vi "Plot Data.vi"(0 "Plots Refnums":T9, 7 "Measurement":T5, 11 "error in (no error)":errorcluster) -> (15 "error out":errorcluster)   [LabVIEW 2014]
uses:
  PlotData Refnums.ctl
  Chooseplot.ctl
  Electrical Data Plot Refnums.ctl
  Optical Spectrum Plot Refnum.ctl
  Measurement.ctl
  WhichInstrument.ctl
  Hardware Control/Parameter Analyzer/Electrical Data.ctl
  Hardware Control/Spectrometer/Spectral Data.ctl
  Hardware Control/Parameter Analyzer/Voltage Plot.ctl
  Hardware Control/Parameter Analyzer/Current Plot.ctl
panel:
  out "PlotData - Choose Plot":T1
  in  "PlotData - Electrical Plot List":T2(tab)
  out "PlotData - Current Plot":cluster{"Time":dbl[], "SMU4":dbl[]}[](graph)=[{"Time"=[0.0, 0.30000000000000004, 0.6000000000000001, 0.9, 1.2000000000000002, 1.5, 1.8, 2.1, 2.4000000000000004, 2.7, 3.0, 3.3000000000000003, 3.6, 3.9000000000000004, 4.2, 4.5, 4.800000000000001, 5.1000000000000005, 5.4, 5.7, 6.0, 6.300000000000001, 6.6000000000000005, 6.9, 7.2, 7.5, 7.800000000000001, 8.1, 8.4, 8.700000000000001, 9.0, 9.3, 9.600000000000001, 9.9, 10.200000000000001, 10.5, 10.8, 11.100000000000001, 11.4, 11.700000000000001, 12.0, 12.3, 12.600000000000001, 12.9, 13.200000000000001, 13.5, 13.8, 14.100000000000001, 14.4, 14.700000000000001, 15.0, 15.3, 15.600000000000001, 15.9, 16.2, 16.5, 16.8, 17.1, 17.400000000000002, 17.7], "SMU4"=[9.99995e-06, 9.99995e-06, 9.99995e-06, 9.99997e-06, 9.99997e-06, 9.99997e-06, 9.99997e-06, 9.999980000000001e-06, 9.99997e-06, 9.999980000000001e-06, 9.99997e-06, 9.999980000000001e-06, 9.99997e-06, 9.99997e-06, 9.99997e-06, 9.99996e-06, 9.99996e-06, 9.99996e-06, 9.99996e-06, 9.99997e-06, 9.99997e-06, 9.999980000000001e-06, 9.99997e-06, 9.99997e-06, 9.99997e-06, 9.99997e-06, 9.99997e-06, 9.999980000000001e-06, 9.999980000000001e-06, 9.99996e-06, 9.99997e-06, 9.99996e-06, 9.99997e-06, 9.99997e-06, 9.99997e-06, 9.99997e-06, 9.999980000000001e-06, 9.99997e-06, 9.999980000000001e-06, 9.999980000000001e-06, 9.99997e-06, 9.99997e-06, 9.99997e-06, 9.99996e-06, 9.99996e-06, 9.99997e-06, 9.99997e-06, 9.99996e-06, 9.99996e-06, 9.99997e-06, 9.99997e-06, 9.99997e-06, 9.99997e-06, 9.99997e-06, 9.99996e-06, 9.99997e-06, 9.99997e-06, 9.99997e-06, 9.99997e-06, 9.99996e-06]}, {"Time"=[0.0, 0.30000000000000004, 0.6000000000000001, 0.9, 1.2000000000000002, 1.5, 1.8, 2.1, 2.4000000000000004, 2.7, 3.0, 3.3000000000000003, 3.6, 3.9000000000000004, 4.2, 4.5, 4.800000000000001, 5.1000000000000005, 5.4, 5.7, 6.0, 6.300000000000001, 6.6000000000000005, 6.9, 7.2, 7.5, 7.800000000000001, 8.1, 8.4, 8.700000000000001, 9.0, 9.3, 9.600000000000001, 9.9, 10.200000000000001, 10.5, 10.8, 11.100000000000001, 11.4, 11.700000000000001, 12.0, 12.3, 12.600000000000001, 12.9, 13.200000000000001, 13.5, 13.8, 14.100000000000001, 14.4, 14.700000000000001, 15.0, 15.3, 15.600000000000001, 15.9, 16.2, 16.5, 16.8, 17.1, 17.400000000000002, 17.7], "SMU4"=[-1.00004e-05, -1.000039e-05, -1.000039e-05, -1.0000409999999999e-05, -1.000039e-05, -1.000039e-05, -1.00004e-05, -1.000043e-05, -1.000042e-05, -1.0000409999999999e-05, -1.000039e-05, -1.000039e-05, -1.0000409999999999e-05, -1.00004e-05, -1.000038e-05, -1.000038e-05, -1.000039e-05, -1.000037e-05, -1.000038e-05, -1.000039e-05, -1.000039e-05, -1.000039e-05, -1.000039e-05, -1.000039e-05, -1.00004e-05, -1.000037e-05, -1.000038e-05, -1.000039e-05, -1.00004e-05, -1.00004e-05, -1.00004e-05, -1.000037e-05, -1.000037e-05, -1.000037e-05, -1.000036e-05, -1.000039e-05, -1.000038e-05, -1.000037e-05, -1.000036e-05, -1.000037e-05, -1.000038e-05, -1.000037e-05, -1.000038e-05, -1.000036e-05, -1.000037e-05, -1.000037e-05, -1.000037e-05, -1.000039e-05, -1.000038e-05, -1.000036e-05, -1.000037e-05, -1.000039e-05, -1.000036e-05, -1.000037e-05, -1.000038e-05, -1.00004e-05, -1.0000409999999999e-05, -1.000038e-05, -1.000038e-05, -1.00004e-05]}]
  out "PlotData - Voltage Plot":cluster{"Time":dbl[], "SMU4":dbl[]}[](graph)=[{"Time"=[0.0, 0.30000000000000004, 0.6000000000000001, 0.9, 1.2000000000000002, 1.5, 1.8, 2.1, 2.4000000000000004, 2.7, 3.0, 3.3000000000000003, 3.6, 3.9000000000000004, 4.2, 4.5, 4.800000000000001, 5.1000000000000005, 5.4, 5.7, 6.0, 6.300000000000001, 6.6000000000000005, 6.9, 7.2, 7.5, 7.800000000000001, 8.1, 8.4, 8.700000000000001, 9.0, 9.3, 9.600000000000001, 9.9, 10.200000000000001, 10.5, 10.8, 11.100000000000001, 11.4, 11.700000000000001, 12.0, 12.3, 12.600000000000001, 12.9, 13.200000000000001, 13.5, 13.8, 14.100000000000001, 14.4, 14.700000000000001, 15.0, 15.3, 15.600000000000001, 15.9, 16.2, 16.5, 16.8, 17.1, 17.400000000000002, 17.7], "SMU4"=[9.99995e-06, 9.99995e-06, 9.99995e-06, 9.99997e-06, 9.99997e-06, 9.99997e-06, 9.99997e-06, 9.999980000000001e-06, 9.99997e-06, 9.999980000000001e-06, 9.99997e-06, 9.999980000000001e-06, 9.99997e-06, 9.99997e-06, 9.99997e-06, 9.99996e-06, 9.99996e-06, 9.99996e-06, 9.99996e-06, 9.99997e-06, 9.99997e-06, 9.999980000000001e-06, 9.99997e-06, 9.99997e-06, 9.99997e-06, 9.99997e-06, 9.99997e-06, 9.999980000000001e-06, 9.999980000000001e-06, 9.99996e-06, 9.99997e-06, 9.99996e-06, 9.99997e-06, 9.99997e-06, 9.99997e-06, 9.99997e-06, 9.999980000000001e-06, 9.99997e-06, 9.999980000000001e-06, 9.999980000000001e-06, 9.99997e-06, 9.99997e-06, 9.99997e-06, 9.99996e-06, 9.99996e-06, 9.99997e-06, 9.99997e-06, 9.99996e-06, 9.99996e-06, 9.99997e-06, 9.99997e-06, 9.99997e-06, 9.99997e-06, 9.99997e-06, 9.99996e-06, 9.99997e-06, 9.99997e-06, 9.99997e-06, 9.99997e-06, 9.99996e-06]}, {"Time"=[0.0, 0.30000000000000004, 0.6000000000000001, 0.9, 1.2000000000000002, 1.5, 1.8, 2.1, 2.4000000000000004, 2.7, 3.0, 3.3000000000000003, 3.6, 3.9000000000000004, 4.2, 4.5, 4.800000000000001, 5.1000000000000005, 5.4, 5.7, 6.0, 6.300000000000001, 6.6000000000000005, 6.9, 7.2, 7.5, 7.800000000000001, 8.1, 8.4, 8.700000000000001, 9.0, 9.3, 9.600000000000001, 9.9, 10.200000000000001, 10.5, 10.8, 11.100000000000001, 11.4, 11.700000000000001, 12.0, 12.3, 12.600000000000001, 12.9, 13.200000000000001, 13.5, 13.8, 14.100000000000001, 14.4, 14.700000000000001, 15.0, 15.3, 15.600000000000001, 15.9, 16.2, 16.5, 16.8, 17.1, 17.400000000000002, 17.7], "SMU4"=[-1.00004e-05, -1.000039e-05, -1.000039e-05, -1.0000409999999999e-05, -1.000039e-05, -1.000039e-05, -1.00004e-05, -1.000043e-05, -1.000042e-05, -1.0000409999999999e-05, -1.000039e-05, -1.000039e-05, -1.0000409999999999e-05, -1.00004e-05, -1.000038e-05, -1.000038e-05, -1.000039e-05, -1.000037e-05, -1.000038e-05, -1.000039e-05, -1.000039e-05, -1.000039e-05, -1.000039e-05, -1.000039e-05, -1.00004e-05, -1.000037e-05, -1.000038e-05, -1.000039e-05, -1.00004e-05, -1.00004e-05, -1.00004e-05, -1.000037e-05, -1.000037e-05, -1.000037e-05, -1.000036e-05, -1.000039e-05, -1.000038e-05, -1.000037e-05, -1.000036e-05, -1.000037e-05, -1.000038e-05, -1.000037e-05, -1.000038e-05, -1.000036e-05, -1.000037e-05, -1.000037e-05, -1.000037e-05, -1.000039e-05, -1.000038e-05, -1.000036e-05, -1.000037e-05, -1.000039e-05, -1.000036e-05, -1.000037e-05, -1.000038e-05, -1.00004e-05, -1.0000409999999999e-05, -1.000038e-05, -1.000038e-05, -1.00004e-05]}]
  out "PlotData - dI/dV-V Characteristic":cluster{"V3":dbl[], "I1":dbl[]}[](graph) caption="Differential Resistance"
  out "PlotData - IV Characteristic":cluster{"V3":dbl[], "I1":dbl[]}[](graph) caption="Current Voltage Characteristic"
  in  "PlotData - Optical Spectra":enum32{"Energy", "Wavelength", "Raman Shift"}(tab)
  out "Optical Spectrum vs Energy":cluster{"data":dbl[], "data":dbl[]}(graph)
  out "Optical Spectrum vs Wavelength":cluster{"data":dbl[], "data":dbl[]}(graph)
  out "Optical Spectrum vs Raman Shift":cluster{"data":dbl[], "data":dbl[]}(graph)
  in  "Optoelectronic Spectrum":enum32{"Energy", "Wavelength", "Raman Shift"}(tab)
  out "Optoelectronic Spectrum vs Energy":cluster{"data":dbl[], "data":dbl[]}(graph)
  out "Optoelectronic Spectrum vs Wavelength":cluster{"data":dbl[], "data":dbl[]}(graph)
  out "Optoelectronic Spectrum vs Raman Shift":cluster{"data":dbl[], "data":dbl[]}(graph)
  out "Optoelectronic Voltage Trace":T3=[{"Time"=[0.0, 0.30000000000000004, 0.6000000000000001, 0.9, 1.2000000000000002, 1.5, 1.8, 2.1, 2.4000000000000004, 2.7, 3.0, 3.3000000000000003, 3.6, 3.9000000000000004, 4.2, 4.5, 4.800000000000001, 5.1000000000000005, 5.4, 5.7, 6.0, 6.300000000000001, 6.6000000000000005, 6.9, 7.2, 7.5, 7.800000000000001, 8.1, 8.4, 8.700000000000001, 9.0, 9.3, 9.600000000000001, 9.9, 10.200000000000001, 10.5, 10.8, 11.100000000000001, 11.4, 11.700000000000001, 12.0, 12.3, 12.600000000000001, 12.9, 13.200000000000001, 13.5, 13.8, 14.100000000000001, 14.4, 14.700000000000001, 15.0, 15.3, 15.600000000000001, 15.9, 16.2, 16.5, 16.8, 17.1, 17.400000000000002, 17.7], "SMU4"=[9.99995e-06, 9.99995e-06, 9.99995e-06, 9.99997e-06, 9.99997e-06, 9.99997e-06, 9.99997e-06, 9.999980000000001e-06, 9.99997e-06, 9.999980000000001e-06, 9.99997e-06, 9.999980000000001e-06, 9.99997e-06, 9.99997e-06, 9.99997e-06, 9.99996e-06, 9.99996e-06, 9.99996e-06, 9.99996e-06, 9.99997e-06, 9.99997e-06, 9.999980000000001e-06, 9.99997e-06, 9.99997e-06, 9.99997e-06, 9.99997e-06, 9.99997e-06, 9.999980000000001e-06, 9.999980000000001e-06, 9.99996e-06, 9.99997e-06, 9.99996e-06, 9.99997e-06, 9.99997e-06, 9.99997e-06, 9.99997e-06, 9.999980000000001e-06, 9.99997e-06, 9.999980000000001e-06, 9.999980000000001e-06, 9.99997e-06, 9.99997e-06, 9.99997e-06, 9.99996e-06, 9.99996e-06, 9.99997e-06, 9.99997e-06, 9.99996e-06, 9.99996e-06, 9.99997e-06, 9.99997e-06, 9.99997e-06, 9.99997e-06, 9.99997e-06, 9.99996e-06, 9.99997e-06, 9.99997e-06, 9.99997e-06, 9.99997e-06, 9.99996e-06]}, {"Time"=[0.0, 0.30000000000000004, 0.6000000000000001, 0.9, 1.2000000000000002, 1.5, 1.8, 2.1, 2.4000000000000004, 2.7, 3.0, 3.3000000000000003, 3.6, 3.9000000000000004, 4.2, 4.5, 4.800000000000001, 5.1000000000000005, 5.4, 5.7, 6.0, 6.300000000000001, 6.6000000000000005, 6.9, 7.2, 7.5, 7.800000000000001, 8.1, 8.4, 8.700000000000001, 9.0, 9.3, 9.600000000000001, 9.9, 10.200000000000001, 10.5, 10.8, 11.100000000000001, 11.4, 11.700000000000001, 12.0, 12.3, 12.600000000000001, 12.9, 13.200000000000001, 13.5, 13.8, 14.100000000000001, 14.4, 14.700000000000001, 15.0, 15.3, 15.600000000000001, 15.9, 16.2, 16.5, 16.8, 17.1, 17.400000000000002, 17.7], "SMU4"=[-1.00004e-05, -1.000039e-05, -1.000039e-05, -1.0000409999999999e-05, -1.000039e-05, -1.000039e-05, -1.00004e-05, -1.000043e-05, -1.000042e-05, -1.0000409999999999e-05, -1.000039e-05, -1.000039e-05, -1.0000409999999999e-05, -1.00004e-05, -1.000038e-05, -1.000038e-05, -1.000039e-05, -1.000037e-05, -1.000038e-05, -1.000039e-05, -1.000039e-05, -1.000039e-05, -1.000039e-05, -1.000039e-05, -1.00004e-05, -1.000037e-05, -1.000038e-05, -1.000039e-05, -1.00004e-05, -1.00004e-05, -1.00004e-05, -1.000037e-05, -1.000037e-05, -1.000037e-05, -1.000036e-05, -1.000039e-05, -1.000038e-05, -1.000037e-05, -1.000036e-05, -1.000037e-05, -1.000038e-05, -1.000037e-05, -1.000038e-05, -1.000036e-05, -1.000037e-05, -1.000037e-05, -1.000037e-05, -1.000039e-05, -1.000038e-05, -1.000036e-05, -1.000037e-05, -1.000039e-05, -1.000036e-05, -1.000037e-05, -1.000038e-05, -1.00004e-05, -1.0000409999999999e-05, -1.000038e-05, -1.000038e-05, -1.00004e-05]}]
  out "Optoelectronic Current Trace":T4=[{"Time"=[0.0, 0.30000000000000004, 0.6000000000000001, 0.9, 1.2000000000000002, 1.5, 1.8, 2.1, 2.4000000000000004, 2.7, 3.0, 3.3000000000000003, 3.6, 3.9000000000000004, 4.2, 4.5, 4.800000000000001, 5.1000000000000005, 5.4, 5.7, 6.0, 6.300000000000001, 6.6000000000000005, 6.9, 7.2, 7.5, 7.800000000000001, 8.1, 8.4, 8.700000000000001, 9.0, 9.3, 9.600000000000001, 9.9, 10.200000000000001, 10.5, 10.8, 11.100000000000001, 11.4, 11.700000000000001, 12.0, 12.3, 12.600000000000001, 12.9, 13.200000000000001, 13.5, 13.8, 14.100000000000001, 14.4, 14.700000000000001, 15.0, 15.3, 15.600000000000001, 15.9, 16.2, 16.5, 16.8, 17.1, 17.400000000000002, 17.7], "SMU4"=[9.99995e-06, 9.99995e-06, 9.99995e-06, 9.99997e-06, 9.99997e-06, 9.99997e-06, 9.99997e-06, 9.999980000000001e-06, 9.99997e-06, 9.999980000000001e-06, 9.99997e-06, 9.999980000000001e-06, 9.99997e-06, 9.99997e-06, 9.99997e-06, 9.99996e-06, 9.99996e-06, 9.99996e-06, 9.99996e-06, 9.99997e-06, 9.99997e-06, 9.999980000000001e-06, 9.99997e-06, 9.99997e-06, 9.99997e-06, 9.99997e-06, 9.99997e-06, 9.999980000000001e-06, 9.999980000000001e-06, 9.99996e-06, 9.99997e-06, 9.99996e-06, 9.99997e-06, 9.99997e-06, 9.99997e-06, 9.99997e-06, 9.999980000000001e-06, 9.99997e-06, 9.999980000000001e-06, 9.999980000000001e-06, 9.99997e-06, 9.99997e-06, 9.99997e-06, 9.99996e-06, 9.99996e-06, 9.99997e-06, 9.99997e-06, 9.99996e-06, 9.99996e-06, 9.99997e-06, 9.99997e-06, 9.99997e-06, 9.99997e-06, 9.99997e-06, 9.99996e-06, 9.99997e-06, 9.99997e-06, 9.99997e-06, 9.99997e-06, 9.99996e-06]}, {"Time"=[0.0, 0.30000000000000004, 0.6000000000000001, 0.9, 1.2000000000000002, 1.5, 1.8, 2.1, 2.4000000000000004, 2.7, 3.0, 3.3000000000000003, 3.6, 3.9000000000000004, 4.2, 4.5, 4.800000000000001, 5.1000000000000005, 5.4, 5.7, 6.0, 6.300000000000001, 6.6000000000000005, 6.9, 7.2, 7.5, 7.800000000000001, 8.1, 8.4, 8.700000000000001, 9.0, 9.3, 9.600000000000001, 9.9, 10.200000000000001, 10.5, 10.8, 11.100000000000001, 11.4, 11.700000000000001, 12.0, 12.3, 12.600000000000001, 12.9, 13.200000000000001, 13.5, 13.8, 14.100000000000001, 14.4, 14.700000000000001, 15.0, 15.3, 15.600000000000001, 15.9, 16.2, 16.5, 16.8, 17.1, 17.400000000000002, 17.7], "SMU4"=[-1.00004e-05, -1.000039e-05, -1.000039e-05, -1.0000409999999999e-05, -1.000039e-05, -1.000039e-05, -1.00004e-05, -1.000043e-05, -1.000042e-05, -1.0000409999999999e-05, -1.000039e-05, -1.000039e-05, -1.0000409999999999e-05, -1.00004e-05, -1.000038e-05, -1.000038e-05, -1.000039e-05, -1.000037e-05, -1.000038e-05, -1.000039e-05, -1.000039e-05, -1.000039e-05, -1.000039e-05, -1.000039e-05, -1.00004e-05, -1.000037e-05, -1.000038e-05, -1.000039e-05, -1.00004e-05, -1.00004e-05, -1.00004e-05, -1.000037e-05, -1.000037e-05, -1.000037e-05, -1.000036e-05, -1.000039e-05, -1.000038e-05, -1.000037e-05, -1.000036e-05, -1.000037e-05, -1.000038e-05, -1.000037e-05, -1.000038e-05, -1.000036e-05, -1.000037e-05, -1.000037e-05, -1.000037e-05, -1.000039e-05, -1.000038e-05, -1.000036e-05, -1.000037e-05, -1.000039e-05, -1.000036e-05, -1.000037e-05, -1.000038e-05, -1.00004e-05, -1.0000409999999999e-05, -1.000038e-05, -1.000038e-05, -1.00004e-05]}]
  # "LICENSED MATERIALS – PROPERTY OF IBM\nCopyright IBM Corp. 2016,\nALL RIGHTS RESERVED"
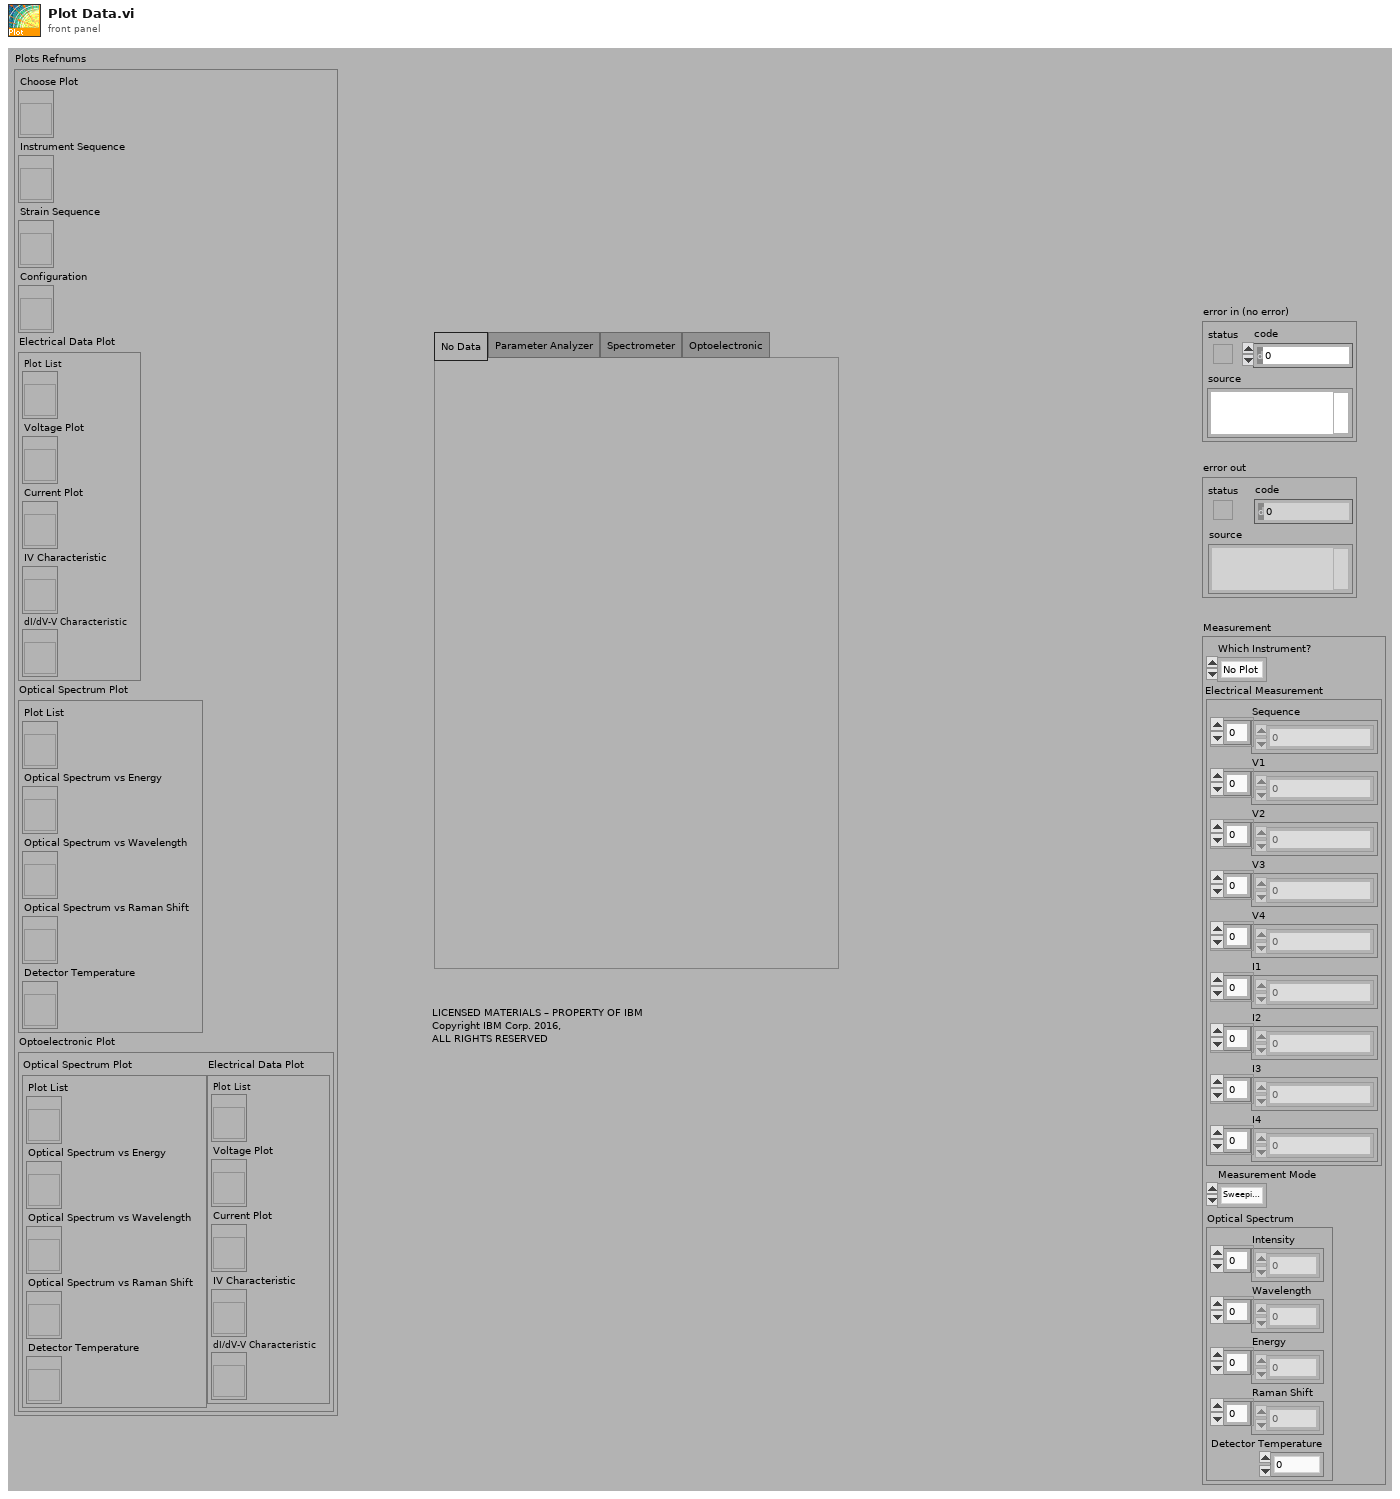
[diagram p1: front panel]
types:
  T1 = typedef "Chooseplot.ctl" = enum32{"No Data", "Parameter Analyzer", "Spectrometer", "Optoelectronic"}
  T2 = enum32{"Current & Voltage Traces", "Four | Two Probe"}
  T3 = typedef "Voltage Plot.ctl" = cluster{"Time":dbl[], "SMU4":dbl[]}[]
  T4 = typedef "Current Plot.ctl" = cluster{"Time":dbl[], "SMU4":dbl[]}[]
  T5 = typedef "Measurement.ctl" = cluster{"Which Instrument?":T6, "Electrical Measurement":T7, "Measurement Mode":enum16{"Sweeping Mode", "Sampling Mode"}, "Optical Spectrum":T8}
  T6 = typedef "WhichInstrument.ctl" = enum16{"No Plot", "Spectrometer", "Parameter Analyzer", "Optoelectronic"}
  T7 = typedef "Electrical Data.ctl" = cluster{"Sequence":dbl[], "V1":dbl[], "V2":dbl[], "V3":dbl[], "V4":dbl[], "I1":dbl[], "I2":dbl[], "I3":dbl[], "I4":dbl[]}
  T8 = typedef "Spectral Data.ctl" = cluster{"Intensity":dbl[], "Wavelength":dbl[], "Energy":dbl[], "Raman Shift":dbl[], "Detector Temperature":dbl}
  T9 = typedef "PlotData Refnums.ctl" = cluster{"Choose Plot":refnum<vi>, "Instrument Sequence":refnum<vi>, "Strain Sequence":refnum<vi>, "Configuration":refnum<vi>, "Electrical Data Plot":T10, "Optical Spectrum Plot":T11, "Optoelectronic Plot":cluster{"Optical Spectrum Plot":T11, "Electrical Data Plot":T10}}
  T10 = typedef "Electrical Data Plot Refnums.ctl" = cluster{"Plot List":refnum<vi>, "Voltage Plot":refnum<vi>, "Current Plot":refnum<vi>, "IV Characteristic":refnum<vi>, "dI/dV-V Characteristic":refnum<vi>}
  T11 = typedef "Optical Spectrum Plot Refnum.ctl" = cluster{"Plot List":refnum<vi>, "Optical Spectrum vs Energy":refnum<vi>, "Optical Spectrum vs Wavelength":refnum<vi>, "Optical Spectrum vs Raman Shift":refnum<vi>, "Detector Temperature":refnum<vi>}
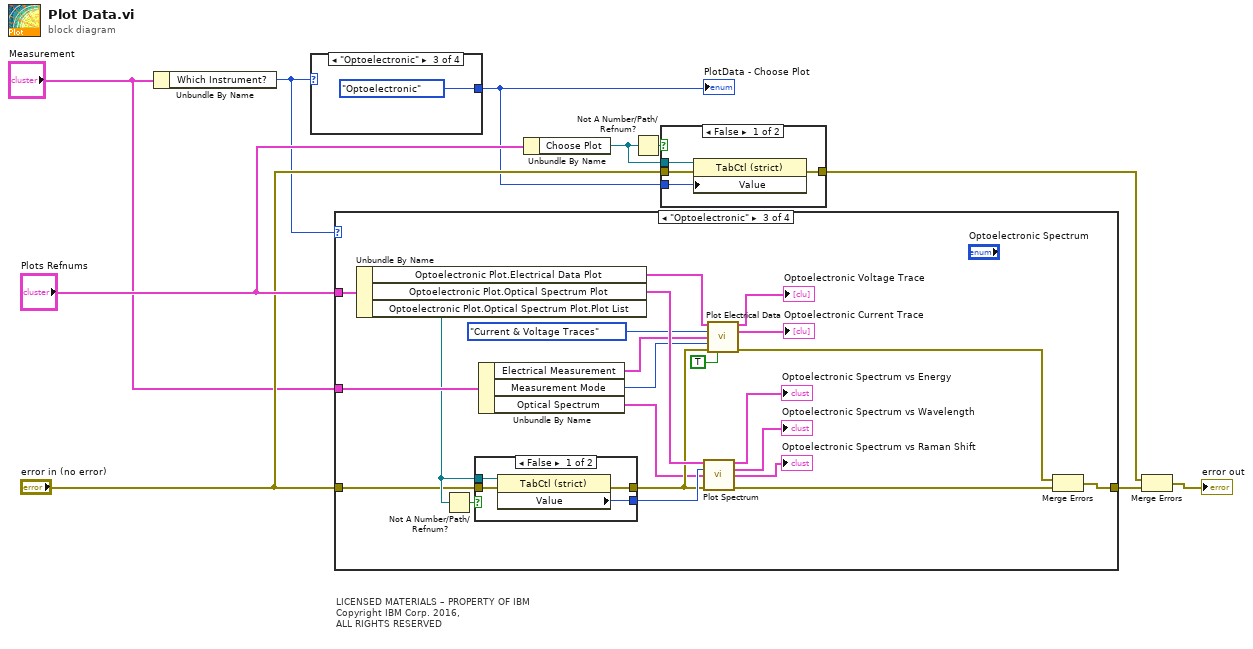
[diagram p0: block diagram]
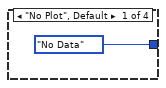
[diagram p2: hidden frame]
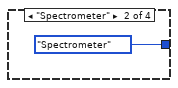
[diagram p3: hidden frame]
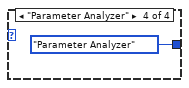
[diagram p4: hidden frame]
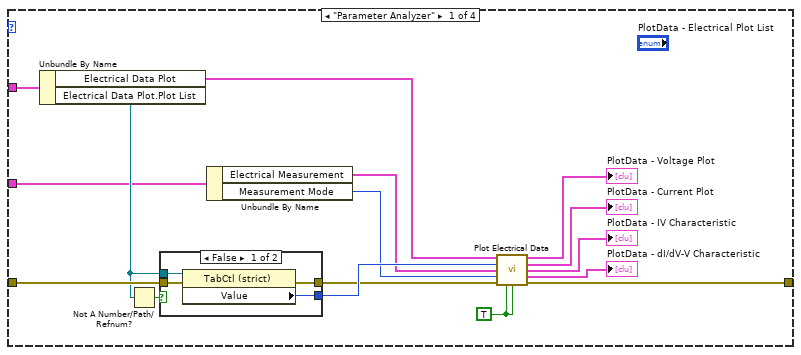
[diagram p6: hidden frame]
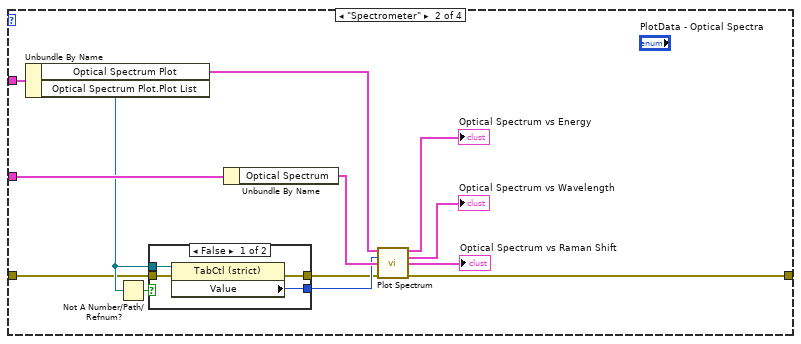
[diagram p8: hidden frame]
diagram:
  # "LICENSED MATERIALS – PROPERTY OF IBM\nCopyright IBM Corp. 2016,\nALL RIGHTS RESERVED"
  n1 = Unbundle By Name("Measurement") -> ("Which Instrument?"=w2:T6)
  n2 = case shown="\"Optoelectronic\"" w2 {
    tunnel: [Chooseplot."No Data" ("PlotData - Choose Plot") Chooseplot."Spectrometer" ("PlotData - Choose Plot") Chooseplot."Optoelectronic" ("PlotData - Choose Plot") Chooseplot."Parameter Analyzer" ("PlotData - Choose Plot")] -> w1
    frame "No Plot", Default {
    }
    frame "Spectrometer" {
    }
    frame "Optoelectronic" {
    }
    frame "Parameter Analyzer" {
    }
  }
  "PlotData - Choose Plot" <- w1
  n3 = case shown="\"Optoelectronic\"" w2 {
    tunnel: [w30 w48 w60 w81] -> w6
    tunnel: "error in (no error)" -> [w26 w40 w69 w81]
    tunnel: "Plots Refnums" -> [w29 w47 w75 _]
    tunnel: "Measurement" -> [w22 w46 w74 _]
    frame "Parameter Analyzer" {
      w19 = TRUE ("Update Pane?")
      n4 = Unbundle By Name(w29) -> ("Electrical Data Plot"=w28:T10, "Electrical Data Plot.Plot List"=w23:refnum<vi>)
      n5 = Not A Number/Path/Refnum?(number/path/refnum=w23) -> (NaN/Path/Refnum?=w24:bool)
      n6 = case shown="False" w24 {
        tunnel: w23 -> [w34 _]
        tunnel: [w33 _] -> w27
        tunnel: w26 -> [w32 w35]
        tunnel: [w31 w35] -> w25
        frame False {
          n7 = property class="TabCtl (strict)"(reference=w34, error in=w32) -> (error out=w31:errorcluster, "Value"=w33:T2)  [unwired: 1 out]
        }
        frame True {
        }
      }
      n8 = Unbundle By Name(w22) -> ("Electrical Measurement"=w21:T7, "Measurement Mode"=w20:enum16{"Sweeping Mode", "Sampling Mode"})
      n9 = call "Plot Electrical Data.vi"("Plot Refnums"=w28, "Plot List"=w27, "Electrical Measurement"=w21, "Measurement Mode"=w20, "error in (no error)"=w25, "Update Labels?"=w19, "Update Pane?"=w19) -> ("Voltage Plot Array"=→"PlotData - Voltage Plot":cluster{"Sequence":dbl[], "Data":dbl[]}[], "Current Plot Array"=→"PlotData - Current Plot":cluster{"Sequence":dbl[], "Data":dbl[]}[], "Current Voltage Array"=→"PlotData - IV Characteristic":cluster{"Voltage":dbl[], "Current":dbl[]}[], "Differential Resistance Array"=→"PlotData - dI/dV-V Characteristic":cluster{"Voltage":dbl[], "Resistance":dbl[]}[], "error out"=w30:errorcluster)  [unwired: 4 out]
    }
    frame "Spectrometer" {
      n10 = Unbundle By Name(w47) -> ("Optical Spectrum Plot"=w44:T11, "Optical Spectrum Plot.Plot List"=w42:refnum<vi>)
      n11 = Not A Number/Path/Refnum?(number/path/refnum=w42) -> (NaN/Path/Refnum?=w43:bool)
      n12 = case shown="False" w43 {
        tunnel: w42 -> [w52 _]
        tunnel: [w51 _] -> w41
        tunnel: w40 -> [w50 w53]
        tunnel: [w49 w53] -> w39
        frame False {
          n13 = property class="TabCtl (strict)"(reference=w52, error in=w50) -> (error out=w49:errorcluster, "Value"=w51:enum32{"Energy", "Wavelength", "Raman Shift"})  [unwired: 1 out]
        }
        frame True {
        }
      }
      n14 = Unbundle By Name(w46) -> ("Optical Spectrum"=w45:T8)
      n15 = call "Plot Spectrum.vi"("Optical Spectrum Plot"=w44, "Optical Spectrum"=w41, "Spectrum"=w45, "error in (no error)"=w39) -> ("Optical Spectrum vs Energy"=→"Optical Spectrum vs Energy":cluster{"data":dbl[], "data":dbl[]}, "Optical Spectrum vs Wavelength"=→"Optical Spectrum vs Wavelength":cluster{"data":dbl[], "data":dbl[]}, "Optical Spectrum vs Raman Shift"=→"Optical Spectrum vs Raman Shift":cluster{"data":dbl[], "data":dbl[]}, "error out"=w48:errorcluster)  [unwired: 8 in]
    }
    frame "Optoelectronic" {
      n16 = Unbundle By Name(w75) -> ("Optoelectronic Plot.Electrical Data Plot"=w62:T10, "Optoelectronic Plot.Optical Spectrum Plot"=w73:T11, "Optoelectronic Plot.Optical Spectrum Plot.Plot List"=w71:refnum<vi>)
      n17 = Not A Number/Path/Refnum?(number/path/refnum=w71) -> (NaN/Path/Refnum?=w72:bool)
      n18 = case shown="False" w72 {
        tunnel: w71 -> [w79 _]
        tunnel: [w78 _] -> w70
        tunnel: w69 -> [w77 w80]
        tunnel: [w76 w80] -> w65
        frame False {
          n19 = property class="TabCtl (strict)"(reference=w79, error in=w77) -> (error out=w76:errorcluster, "Value"=w78:enum32{"Energy", "Wavelength", "Raman Shift"})  [unwired: 1 out]
        }
        frame True {
        }
      }
      n20 = Unbundle By Name(w74) -> ("Electrical Measurement"=w57:T7, "Measurement Mode"=w55:enum16{"Sweeping Mode", "Sampling Mode"}, "Optical Spectrum"=w56:T8)
      n21 = call "Plot Spectrum.vi"("Optical Spectrum Plot"=w73, "Optical Spectrum"=w70, "Spectrum"=w56, "error in (no error)"=w65) -> ("Optical Spectrum vs Energy"=→"Optoelectronic Spectrum vs Energy":cluster{"data":dbl[], "data":dbl[]}, "Optical Spectrum vs Wavelength"=→"Optoelectronic Spectrum vs Wavelength":cluster{"data":dbl[], "data":dbl[]}, "Optical Spectrum vs Raman Shift"=→"Optoelectronic Spectrum vs Raman Shift":cluster{"data":dbl[], "data":dbl[]}, "error out"=w61:errorcluster)  [unwired: 8 in]
      n22 = call "Plot Electrical Data.vi"("Plot Refnums"=w62, "Plot List"=T2."Current & Voltage Traces", "Electrical Measurement"=w57, "Measurement Mode"=w55, "error in (no error)"=w65, "Update Labels?"=TRUE) -> ("Voltage Plot Array"=→"Optoelectronic Voltage Trace":cluster{"Sequence":dbl[], "Data":dbl[]}[], "Current Plot Array"=→"Optoelectronic Current Trace":cluster{"Sequence":dbl[], "Data":dbl[]}[], "error out"=w59:errorcluster)  [unwired: 1 in, 6 out]
      n23 = Merge Errors(w59, w61) -> (w60:errorcluster)
    }
    frame "No Plot", Default {
    }
  }
  n24 = Unbundle By Name("Plots Refnums") -> ("Choose Plot"=w4:refnum<vi>)
  n25 = Not A Number/Path/Refnum?(number/path/refnum=w4) -> (NaN/Path/Refnum?=w5:bool)
  n26 = case shown="False" w5 {
    tunnel: w4 -> [w85 _]
    tunnel: "error in (no error)" -> [w84 w86]
    tunnel: [w83 w86] -> w7
    tunnel: w1 -> [w82 _]
    frame False {
      n27 = property class="TabCtl (strict)"(reference=w85, error in=w84, "Value"=w82) -> (error out=w83:errorcluster)  [unwired: 1 out]
    }
    frame True {
    }
  }
  n28 = Merge Errors(w7, w6) -> (→"error out":errorcluster)
